vi "Periodic Tasks.vi"(8 "error constant":errorcluster) -> ()   [LabVIEW 2019]
doc: "This VI runs in parallel to other tasks. It can contain as many user-defined periodic loops as you need. These can carry out PID or other sorts of timed response."
uses:
  Vanna/Vanna Global.vi
  Drive/Drive Global.vi
  Climb/Climb Global.vi
  Shoot/Shoot Global.vi
  <vilib>/Rock Robotics/Network Tables/NT Write Variant.vi
  Calculations or utilities/Is command done typedef.ctl
panel:
  in  "Commands":T2
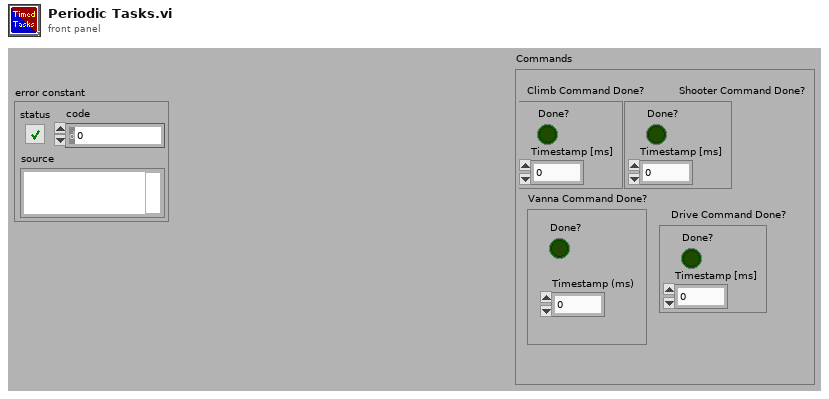
[diagram p1: front panel]
types:
  T1 = typedef "Is command done typedef.ctl" = cluster{"Done?":bool, "Timestamp [ms]":dbl}
  T2 = cluster{"Climb Command Done?":T1, "Shooter Command Done?":T1, "Vanna Command Done?":cluster{"Done?":bool, "Timestamp (ms)":dbl}, "Drive Command Done?":T1}
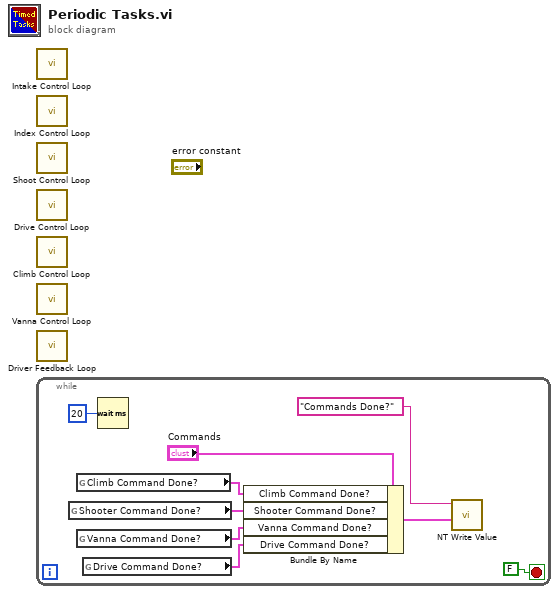
[diagram p0: block diagram]
diagram:
  n1 = call "Intake Control Loop.vi"() -> ()  [unwired: 12 in]
  n2 = call "Index Control Loop.vi"() -> ()  [unwired: 12 in]
  n3 = call "Shoot Control Loop.vi"() -> ()  [unwired: 12 in]
  n4 = call "Drive Control Loop.vi"() -> ()  [unwired: 12 in]
  n5 = call "Climb Control Loop.vi"() -> ()  [unwired: 12 in]
  n6 = call "Vanna Control Loop.vi"() -> ()  [unwired: 12 in]
  n7 = call "Driver Feedback Loop.vi"() -> ()  [unwired: 12 in]
  n8 = while {
    stop <- FALSE stop-if-true
    n9 = global read "Shoot Global.vi" "Shooter Command Done?"() -> (w5:T1)
    n10 = global read "Climb Global.vi" "Climb Command Done?"() -> (w6:T1)
    n11 = global read "Vanna Global.vi" "Vanna Command Done?"() -> (w4:cluster{"Done?":bool, "Timestamp (ms)":dbl})
    n12 = global read "Drive Global.vi" "Drive Command Done?"() -> (w3:T1)
    n13 = Wait (ms)(milliseconds to wait=u32 20 ("millisecond timer value")) -> ()  [unwired: 1 out]
    n14 = Bundle By Name(cluster="Commands", "Climb Command Done?"=w6, "Shooter Command Done?"=w5, "Vanna Command Done?"=w4, "Drive Command Done?"=w3) -> (w2:T2)
    n15 = call-poly <vilib>:"NT Write Value.vi"("Variant"=w2, "Name"="Commands Done?") -> ()  [unwired: 9 in, 1 out]
  }
